vi "testLowLevelSocketConnection.vi"() -> ()   [LabVIEW 2012]
uses:
  <vilib>/Utility/NIReport.llb/NI_report.lvclass
  <vilib>/Utility/NIReport.llb/HTML/NI_HTML.lvclass
panel:
  in  "Att_en_b":bool=TRUE
  in  "Ib_ClipVb":u32=63
  in  "Clip_en_b":bool=TRUE
  in  "CompBuf_en_b":bool
  in  "Att gain":u32
  in  "Clip_sel_b":u32=1
  out "Register Select":string="10@5-3_0\r\n"
  in  "Channel":i32
  in  "Action":i32=3
  out "Data Write":string="8255@6-3_0\r\n"
  out "Data":i32=8255
  in  "Instrument VISA in":T1={"AWG VISA"="AgilentGenerator1", "Oscilloscope  VISA "="AgilentOsciloscope", "Integration Board IP"="172.16.17.47", "connection ID"=refnum, "report out"=refnum, "report file path"=path "C:/Documents and Settings/CTA_LAB01/Desktop/L0_Asic/L0 Asic Test Data"}
  out "error out":errorcluster
  in  "error in":errorcluster
  # "8703"
  # "8511"
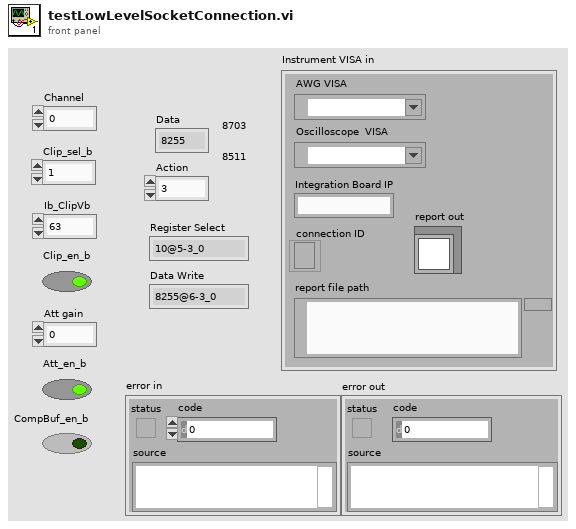
[diagram p1: front panel]
types:
  T1 = cluster{"AWG VISA":refnum<visa-resource-name>, "Oscilloscope  VISA ":refnum<visa-resource-name>, "Integration Board IP":string, "connection ID":refnum<k5>, "report out":refnum<class "NI_report.lvclass">, "report file path":path}
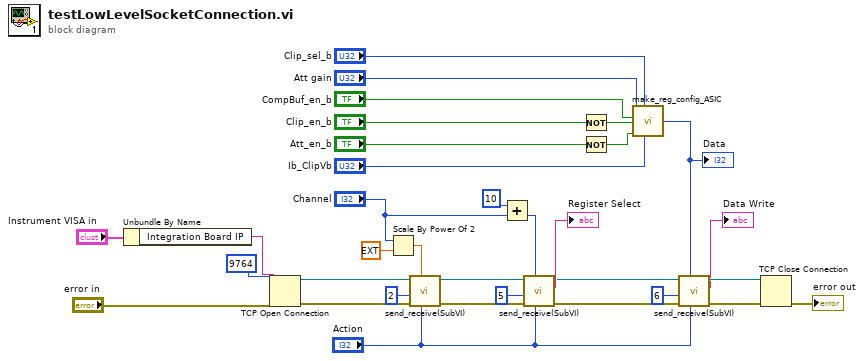
[diagram p0: block diagram]
diagram:
  n1 = Unbundle By Name("Instrument VISA in") -> ("Integration Board IP"=w30:string)
  n2 = TCP Open Connection(address=w30, remote port or service name=9764, error in (no error)="error in") -> (connection ID=w8:refnum<k5>, error out=w10:errorcluster)  [unwired: 2 in]
  n3 = Scale By Power Of 2(n="Channel", x=ext 1.0) -> (x*2^n=w1:ext)
  n4 = call "send_receive(SubVI).vi"("Action"="Action", "Data"=w1, "error in"=w10, "Address"=2, "connection ID"=w8) -> ("error out"=w9:errorcluster, "connection ID out"=w7:refnum<k5>)  [unwired: 2 in, 3 out]
  n5 = Add(x=10, y="Channel") -> (x+y=w14:i32)
  n6 = call "send_receive(SubVI).vi"("Action"="Action", "Data"=w14, "error in"=w9, "Address"=5, "connection ID"=w7) -> ("error out"=w24:errorcluster, "connection ID out"=w5:refnum<k5>, "data in"=→"Register Select":string)  [unwired: 2 in, 2 out]
  n7 = Not(x="Clip_en_b") -> (.not. x?=w11:bool)
  n8 = Not(x="Att_en_b") -> (.not. x?=w12:bool)
  n9 = call "make_reg_config_ASIC.vi"("Ib_ClipVb"="Ib_ClipVb", "Clip_sel_b"="Clip_sel_b", "Att_en_b"=w12, "Clip_en_b"=w11, "CompBuf_en_b"="CompBuf_en_b", "Att gain"="Att gain") -> ("Out reg value"=w21:u32)
  "Data" <- w21
  n10 = call "send_receive(SubVI).vi"("Action"="Action", "Data"=w21, "error in"=w24, "Address"=6, "connection ID"=w5) -> ("error out"=w28:errorcluster, "connection ID out"=w27:refnum<k5>, "data in"=→"Data Write":string)  [unwired: 2 in, 2 out]
  n11 = TCP Close Connection(connection ID=w27, error in (no error)=w28) -> (error out=→"error out":errorcluster)  [unwired: 1 in, 1 out]
